vi "SMU_gate_2_sweep.vi"() -> ()   [LabVIEW 2022 SP3]
uses:
  Agilent U2722/Public/Configure/Configure Channel (Current).vi
  <vilib>/Analysis/1siggen.llb/Ramp Pattern by Delta.vi
  Agilent U2722/Public/Configure/Configure Channel (Voltage).vi
  Agilent U2722/Public/Data/Read Output (Single).vi
  <vilib>/Utility/file.llb/Write Delimited Spreadsheet (DBL).vi
  Agilent U2722/Agilent U2722.lvlib
  <vilib>/Analysis/NI_AALBase.lvlib
panel:
  in  "Tab Control":enum32{"Device Setup"}(tab)
  in  "OK Button":bool
  in  "Select Waveform":u16(ring) items=["Constant", "Sweep", "Pulse"]
  out "Vdd (V)":dbl
  in  "Voltage Range 2":u16(ring) items=["2 Volts", "20 Volts"]
  in  "Current Range 2":u16(ring)=4 items=["1 uA", "10 uA", "100 uA", "1 mA", "10 mA", "120 mA"]
  in  "Current Limit  2":dbl=0.005 format="%#_2p"
  in  "Voltage Range":u16(ring) items=["2 Volts", "20 Volts"]
  in  "Starting Voltage (V)":dbl
  in  "Stopping Voltage (V)":dbl=1.0
  in  "Voltage Interval  (DV)":dbl format="%#_2g"
  in  "Current Range":u16(ring)=4 items=["1 uA", "10 uA", "100 uA", "1 mA", "10 mA", "120 mA"]
  in  "VISA resource name SMU 1":refnum<visa-resource-name>
  in  "Gate 1 Channel Config":u16(ring)=1 items=["Channel 1"=1, "Channel 2"=2, "Channel 3"=3]
  in  "PLC":i32
  in  "Current Limit":dbl=0.005 format="%#_2p"
  in  "Interval Time (s)":dbl=1.0 caption="Delay Time (s)"
  in  "Vdd Channel Config":u16(ring)=2 items=["Channel 1"=1, "Channel 2"=2, "Channel 3"=3]
  in  "output file path":path
  out "XY Graph":cluster{"Y":dbl[], "Y":dbl[]}[](graph)
  in  "VISA resource name SMU 2":refnum<visa-resource-name>
  in  "Voltage Range 3":u16(ring) items=["2 Volts", "20 Volts"]
  in  "Current Range 3":u16(ring)=4 items=["1 uA", "10 uA", "100 uA", "1 mA", "10 mA", "120 mA"]
  in  "Gate 2 Channel Config":u16(ring)=1 items=["Channel 1"=1, "Channel 2"=2, "Channel 3"=3]
  in  "PLC 2":i32
  in  "Current Limit  3":dbl=0.005 format="%#_2p"
  in  "Output Measure Channel Config":u16(ring)=2 items=["Channel 1"=1, "Channel 2"=2, "Channel 3"=3]
  out "Idd (A)":dbl
  in  "Starting Voltage (V)":dbl
  in  "Stopping Voltage (V)":dbl=1.0
  in  "Voltage Interval  (DV)":dbl format="%#_2g"
  in  "Gate 2 Voltage (V)":dbl
  out "I_gate2 (A)":dbl
  out "V_gate2 (V)":dbl
  out "V_gate1 (A)":dbl
  out "I_gate1 (A)":dbl
  in  "Gate 1 Voltage (V)":dbl
  in  "Select Waveform":u16(ring) items=["Constant", "Sweep", "Pulse"]
  in  "Vdd (V) 2":dbl
  in  "Voltage Interval  (DV)":dbl format="%#_2g"
  in  "Stopping Voltage (V)":dbl=1.0
  in  "Starting Voltage (V)":dbl
  in  "Select Waveform":u16(ring) items=["Constant", "Sweep", "Pulse"]
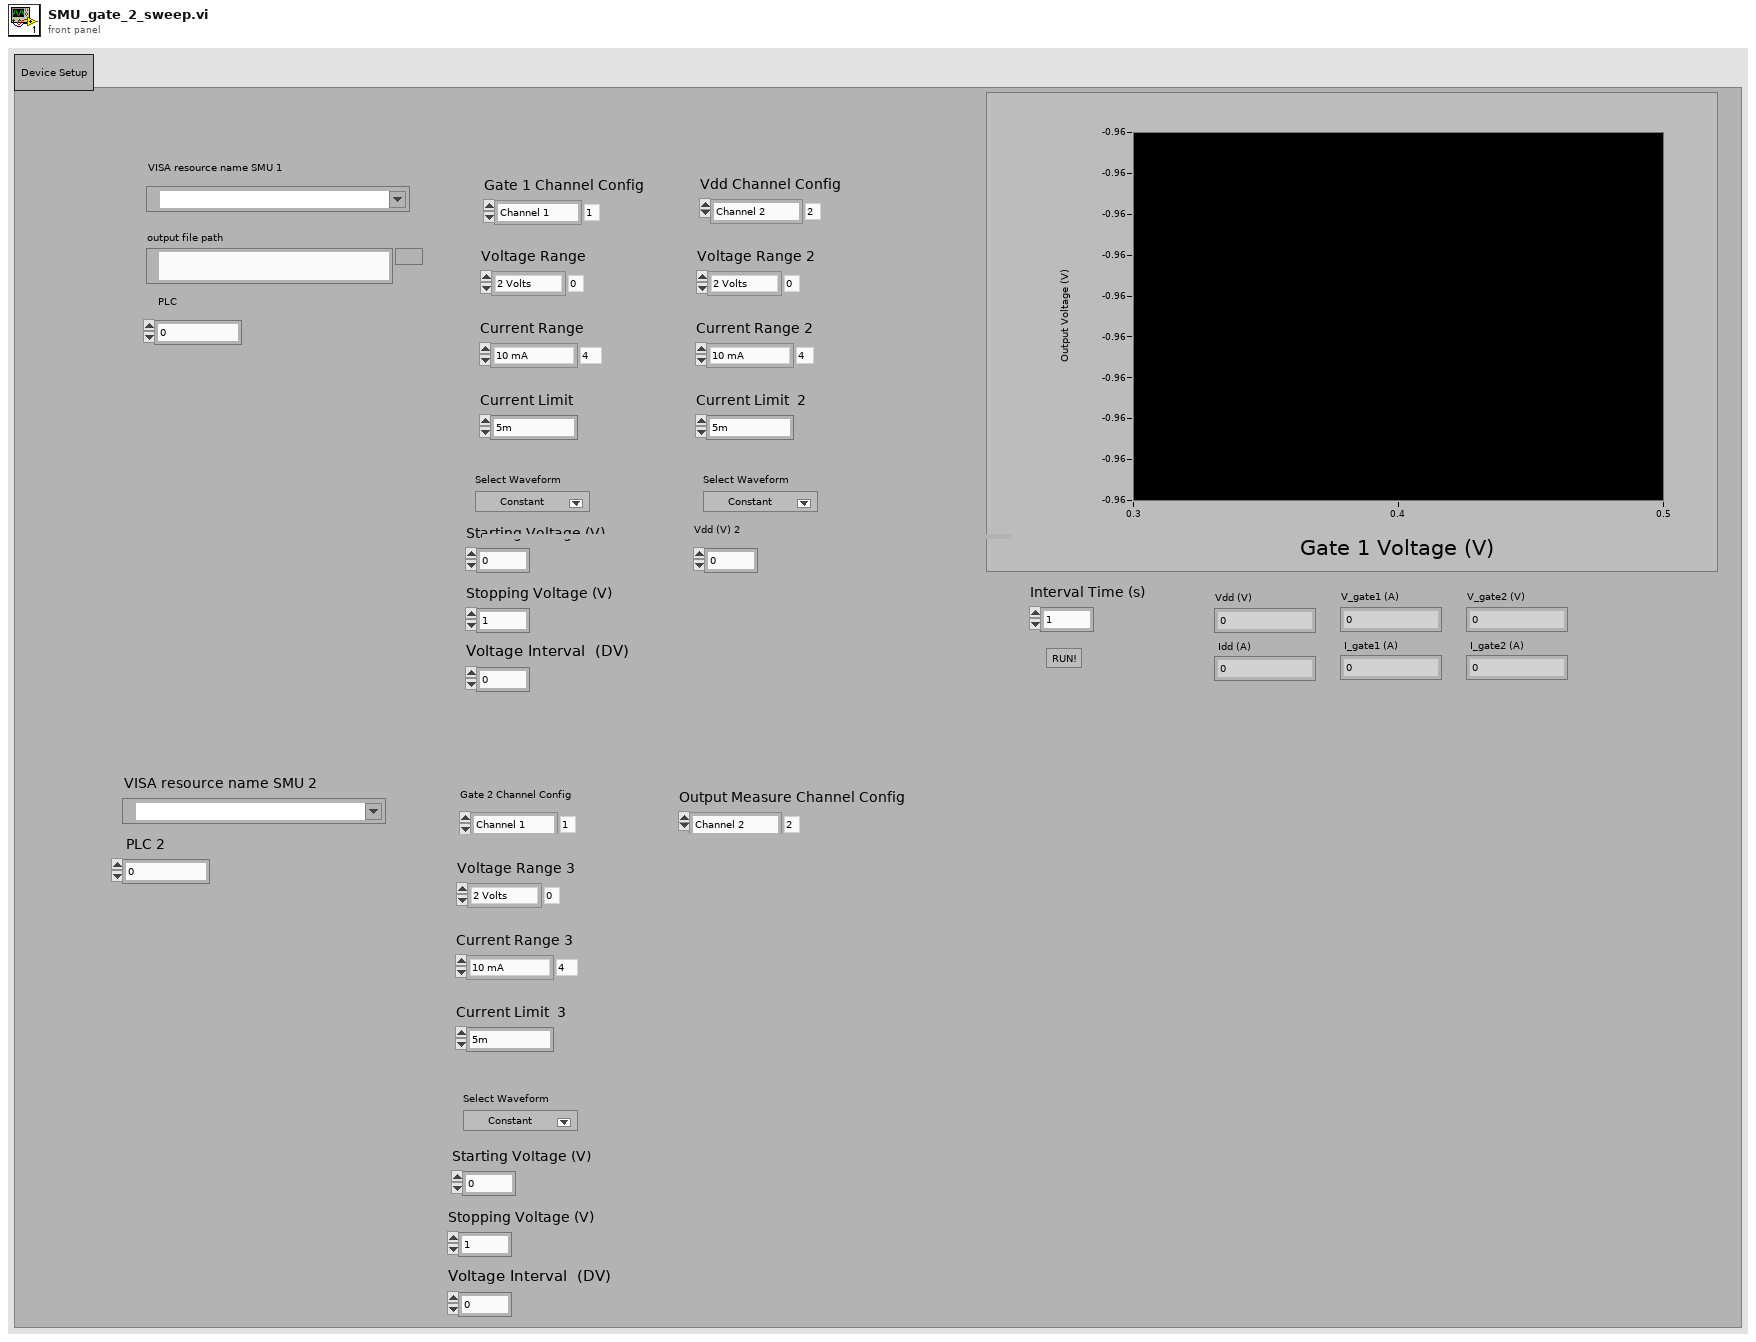
[diagram p1: front panel]
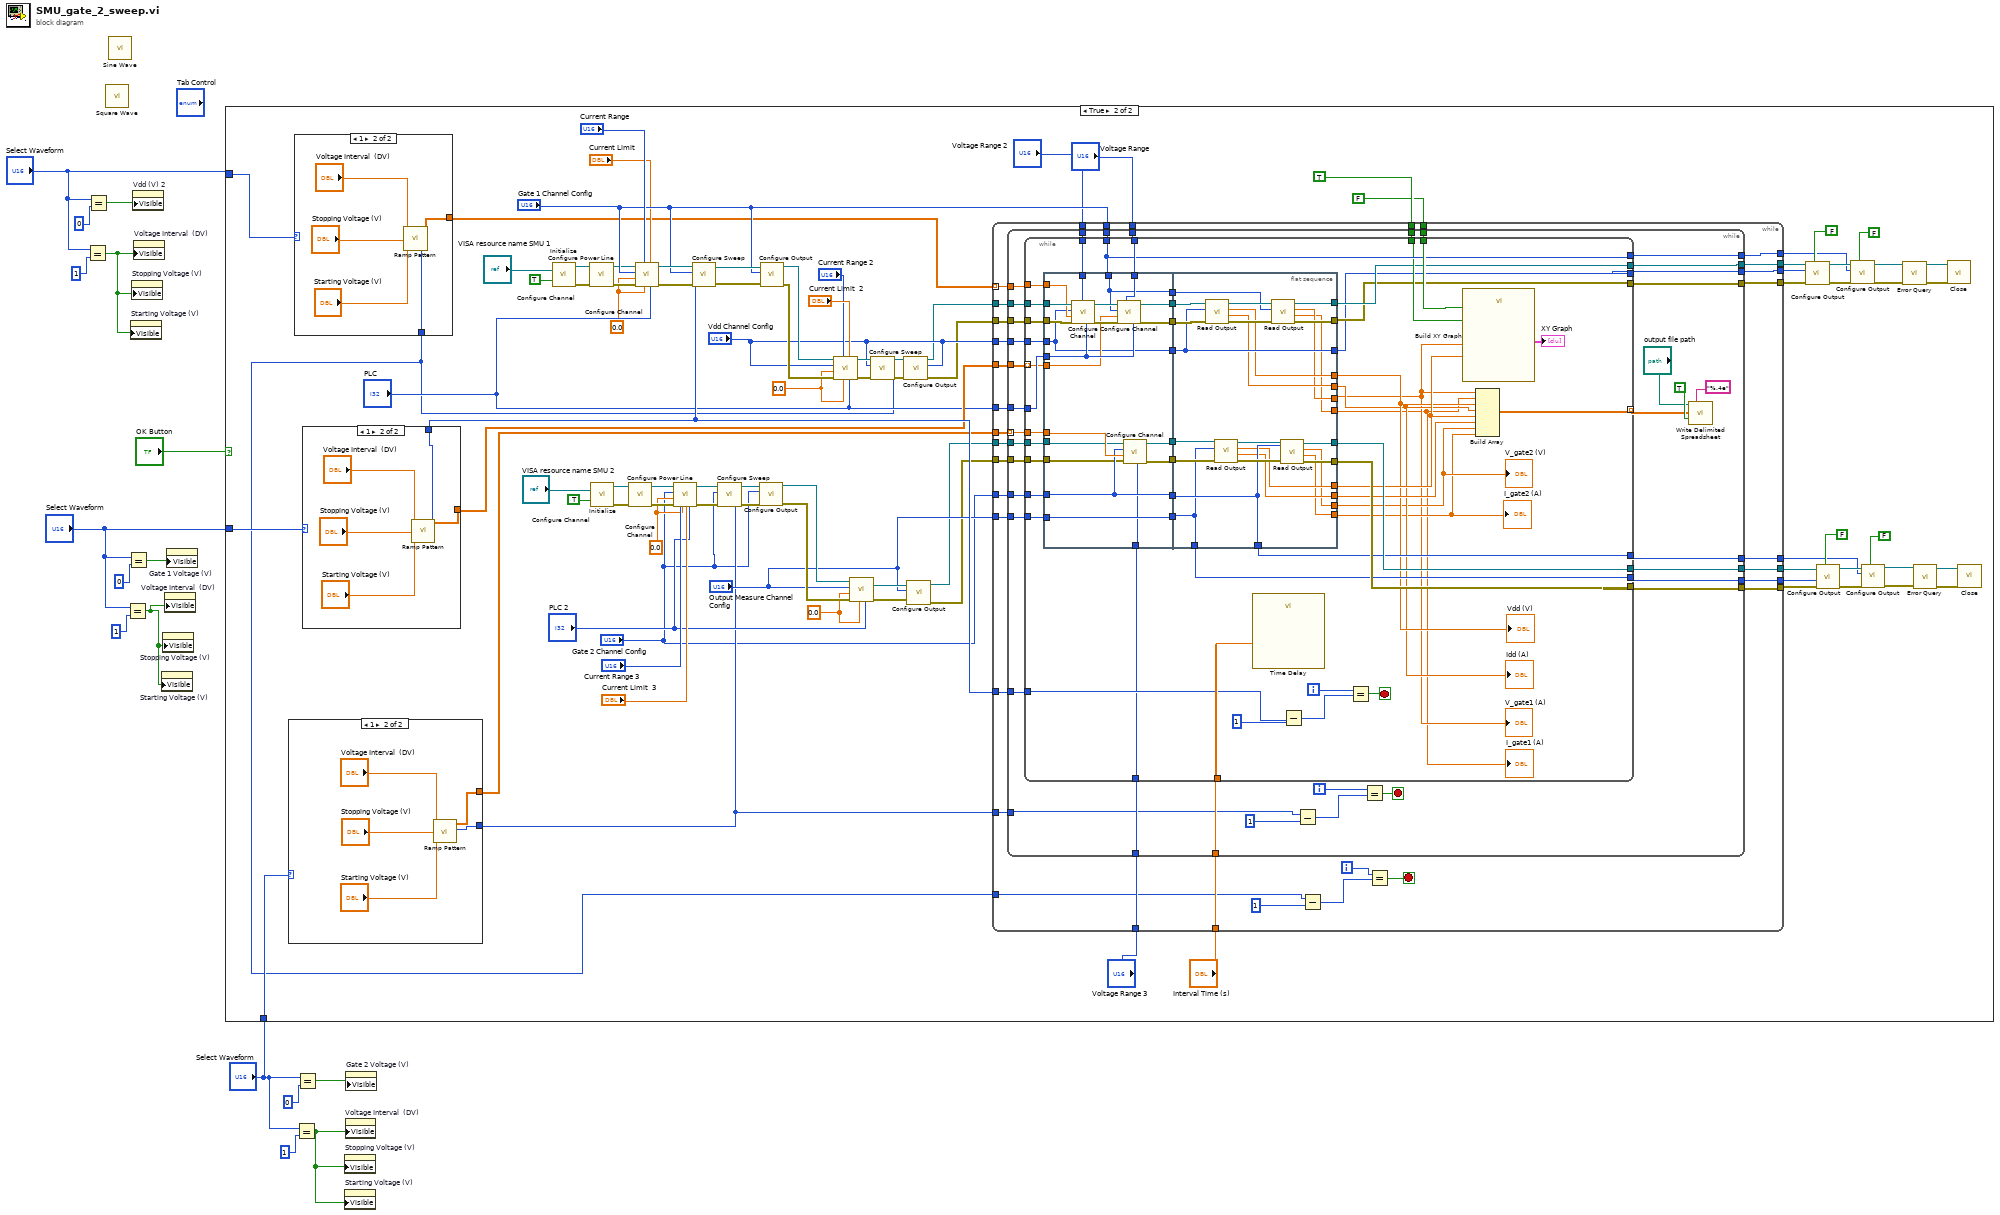
[diagram p0: block diagram]
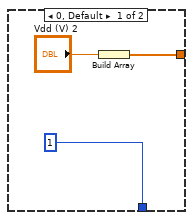
[diagram p3: hidden frame]
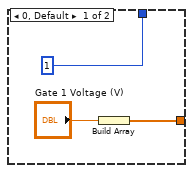
[diagram p4: hidden frame]
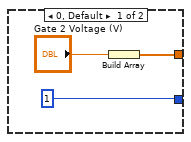
[diagram p5: hidden frame]
diagram:
  n1 = Equal?(x="Select Waveform", y=1) -> (x = y?=w3:bool)
  n2 = Equal?(x="Select Waveform", y=0) -> (x = y?=w2:bool)
  n3 = call <vilib>:"Square Wave.vi"() -> ()  [unwired: 6 in, 3 out]
  n4 = call <vilib>:"Sine Wave.vi"() -> ()  [unwired: 5 in, 3 out]
  n5 = Equal?(x="Select Waveform", y=1) -> (x = y?=w6:bool)
  n6 = Equal?(x="Select Waveform", y=0) -> (x = y?=w7:bool)
  n7 = property on="Starting Voltage (V)" class="DigNum (strict)"("Visible"=w3) -> ()  [unwired: 2 in, 2 out]
  n8 = property on="Stopping Voltage (V)" class="DigNum (strict)"("Visible"=w3) -> ()  [unwired: 2 in, 2 out]
  n9 = property on="Vdd (V) 2" class="DigNum (strict)"("Visible"=w2) -> ()  [unwired: 2 in, 2 out]
  n10 = property on="Voltage Interval  (DV)" class="DigNum (strict)"("Visible"=w3) -> ()  [unwired: 2 in, 2 out]
  n11 = property on="Starting Voltage (V)" class="DigNum (strict)"("Visible"=w6) -> ()  [unwired: 2 in, 2 out]
  n12 = property on="Stopping Voltage (V)" class="DigNum (strict)"("Visible"=w6) -> ()  [unwired: 2 in, 2 out]
  n13 = property on="Voltage Interval  (DV)" class="DigNum (strict)"("Visible"=w6) -> ()  [unwired: 2 in, 2 out]
  n14 = property on="Gate 1 Voltage (V)" class="DigNum (strict)"("Visible"=w7) -> ()  [unwired: 2 in, 2 out]
  n15 = case shown="True" "OK Button" {
    tunnel: "Select Waveform" -> [_ w38]
    tunnel: "Select Waveform" -> [_ w34]
    tunnel: "Select Waveform" -> [_ w33]
    frame False {
    }
    frame True {
      w58 = 0.0
      w57 = 0.0
      w71 = 0.0
      w70 = 0.0
      n16 = case shown="1" w38 {
        tunnel: [w285 w288] -> w37
        tunnel: [1 w287] -> w35
        frame 0, Default {
          n17 = Build Array("Gate 2 Voltage (V)") -> (w285:dbl[])
        }
        frame 1 {
          n18 = call-poly <vilib>:"Ramp Pattern.vi"("start"="Starting Voltage (V)", "end"="Stopping Voltage (V)", "delta"="Voltage Interval  (DV)") -> ("samples"=w287:i32, "Ramp Pattern"=w288:dbl[])  [unwired: 6 in, 1 out]
        }
      }
      n19 = case shown="1" w33 {
        tunnel: [1 w272] -> w26
        tunnel: [w268 w271] -> w28
        frame 0, Default {
          n20 = Build Array("Vdd (V) 2") -> (w268:dbl[])
        }
        frame 1 {
          n21 = call-poly <vilib>:"Ramp Pattern.vi"("start"="Starting Voltage (V)", "end"="Stopping Voltage (V)", "delta"="Voltage Interval  (DV)") -> ("samples"=w272:i32, "Ramp Pattern"=w271:dbl[])  [unwired: 6 in, 1 out]
        }
      }
      n22 = case shown="1" w34 {
        tunnel: [1 w280] -> w93
        tunnel: [w276 w279] -> w87
        frame 0, Default {
          n23 = Build Array("Gate 1 Voltage (V)") -> (w276:dbl[])
        }
        frame 1 {
          n24 = call-poly <vilib>:"Ramp Pattern.vi"("start"="Starting Voltage (V)", "end"="Stopping Voltage (V)", "delta"="Voltage Interval  (DV)") -> ("samples"=w280:i32, "Ramp Pattern"=w279:dbl[])  [unwired: 6 in, 1 out]
        }
      }
      n25 = call "Initialize.vi"("ID Query (True)"=TRUE, "VISA resource name"="VISA resource name SMU 1") -> ("error out"=w103:errorcluster, "VISA resource name out"=w102:refnum<visa-resource-name>)  [unwired: 8 in]
      n26 = call "Configure Power Line.vi"("error in (no error)"=w103, "VISA resource name"=w102) -> ("error out"=w89:errorcluster, "VISA resource name out"=w85:refnum<visa-resource-name>)  [unwired: 8 in]
      n27 = call "Initialize.vi"("ID Query (True)"=TRUE, "VISA resource name"="VISA resource name SMU 2") -> ("error out"=w66:errorcluster, "VISA resource name out"=w65:refnum<visa-resource-name>)  [unwired: 8 in]
      n28 = call "Configure Power Line.vi"("error in (no error)"=w66, "VISA resource name"=w65) -> ("error out"=w64:errorcluster, "VISA resource name out"=w62:refnum<visa-resource-name>)  [unwired: 8 in]
      n29 = call-poly "Configure Channel.vi"("Power Line Cycles (0)"="PLC", "Current Limit (1.0 uA)"="Current Limit", "Triggered Level (1.0 mA)"=w70, "Current Range (0: 1 uA)"="Current Range", "error in (no error)"=w89, "Output Level (1.0 mA)"=w70, "Channel (1: Channel 1)"="Gate 1 Channel Config", "VISA resource name"=w85) -> ("error out"=w90:errorcluster, "VISA resource name out"=w91:refnum<visa-resource-name>)  [unwired: 2 in]
      n30 = call-poly "Configure Channel.vi"("Power Line Cycles (0)"="PLC 2", "Current Limit (1.0 uA)"="Current Limit  3", "Triggered Level (1.0 mA)"=w57, "Current Range (0: 1 uA)"="Current Range 3", "error in (no error)"=w64, "Output Level (1.0 mA)"=w57, "Channel (1: Channel 1)"="Gate 2 Channel Config", "VISA resource name"=w62) -> ("error out"=w41:errorcluster, "VISA resource name out"=w42:refnum<visa-resource-name>)  [unwired: 2 in]
      n31 = call "Configure Sweep.vi"("error in (no error)"=w90, "Sweep Points (1)"=w93, "Channel (1: Channel 1)"="Gate 1 Channel Config", "VISA resource name"=w91) -> ("error out"=w94:errorcluster, "VISA resource name out"=w95:refnum<visa-resource-name>)  [unwired: 6 in]
      n32 = call "Configure Sweep.vi"("error in (no error)"=w41, "Sweep Points (1)"=w35, "Channel (1: Channel 1)"="Gate 2 Channel Config", "VISA resource name"=w42) -> ("error out"=w39:errorcluster, "VISA resource name out"=w40:refnum<visa-resource-name>)  [unwired: 6 in]
      n33 = call "Configure Output.vi"("error in (no error)"=w39, "Channel (1: Channel 1)"="Gate 2 Channel Config", "VISA resource name"=w40) -> ("error out"=w60:errorcluster, "VISA resource name out"=w61:refnum<visa-resource-name>)  [unwired: 7 in]
      n34 = call "Configure Output.vi"("error in (no error)"=w94, "Channel (1: Channel 1)"="Gate 1 Channel Config", "VISA resource name"=w95) -> ("error out"=w83:errorcluster, "VISA resource name out"=w84:refnum<visa-resource-name>)  [unwired: 7 in]
      n35 = call-poly "Configure Channel.vi"("Power Line Cycles (0)"="PLC", "Current Limit (1.0 uA)"="Current Limit  2", "Triggered Level (1.0 mA)"=w71, "Current Range (0: 1 uA)"="Current Range 2", "error in (no error)"=w83, "Output Level (1.0 mA)"=w71, "Channel (1: Channel 1)"="Vdd Channel Config", "VISA resource name"=w84) -> ("error out"=w29:errorcluster, "VISA resource name out"=w32:refnum<visa-resource-name>)  [unwired: 2 in]
      n36 = call-poly "Configure Channel.vi"("Power Line Cycles (0)"="PLC 2", "Triggered Level (1.0 mA)"=w58, "error in (no error)"=w60, "Output Level (1.0 mA)"=w58, "Channel (1: Channel 1)"="Output Measure Channel Config", "VISA resource name"=w61) -> ("error out"=w55:errorcluster, "VISA resource name out"=w56:refnum<visa-resource-name>)  [unwired: 4 in]
      n37 = call "Configure Sweep.vi"("error in (no error)"=w29, "Sweep Points (1)"=w26, "Channel (1: Channel 1)"="Vdd Channel Config", "VISA resource name"=w32) -> ("error out"=w30:errorcluster, "VISA resource name out"=w31:refnum<visa-resource-name>)  [unwired: 6 in]
      n38 = call "Configure Output.vi"("error in (no error)"=w30, "Channel (1: Channel 1)"="Vdd Channel Config", "VISA resource name"=w31) -> ("error out"=w25:errorcluster, "VISA resource name out"=w24:refnum<visa-resource-name>)  [unwired: 7 in]
      n39 = call "Configure Output.vi"("error in (no error)"=w55, "Channel (1: Channel 1)"="Output Measure Channel Config", "VISA resource name"=w56) -> ("error out"=w19:errorcluster, "VISA resource name out"=w20:refnum<visa-resource-name>)  [unwired: 7 in]
      n40 = while {
        tunnel: TRUE -> [w138]
        tunnel: FALSE -> [w137]
        tunnel: "Interval Time (s)" -> [w136]
        tunnel: w93 -> [w135]
        tunnel: "Voltage Range" -> [w134]
        tunnel: w87 -> [w133]
        tunnel: "Gate 1 Channel Config" -> [w132]
        tunnel: [w131] -> w77
        tunnel: [w130] -> w76
        tunnel: "PLC" -> [w129]
        tunnel: "Voltage Range 2" -> [w128]
        tunnel: "Output Measure Channel Config" -> [w127]
        tunnel: [w126] -> w45
        tunnel: [w125] -> w44
        tunnel: "Voltage Range 3" -> [w124]
        tunnel: w37 -> [w123]
        tunnel: w35 -> [w122]
        tunnel: "Gate 2 Channel Config" -> [w121]
        tunnel: w28 -> [w120] mode=indexing
        tunnel: "Vdd Channel Config" -> [w119]
        tunnel: w26 -> [w115]
        tunnel: w25 -> [w113]
        tunnel: w24 -> [w112]
        tunnel: [w111] -> w23
        tunnel: [w110] -> w22
        tunnel: w20 -> [w109]
        tunnel: w19 -> [w108]
        tunnel: [w107] -> w18
        tunnel: [w106] -> w17
        i -> [w116]
        stop <- w114 stop-if-true
        n41 = while {
          tunnel: w138 -> [w174]
          tunnel: w137 -> [w173]
          tunnel: w136 -> [w172]
          tunnel: w135 -> [w171]
          tunnel: w134 -> [w170]
          tunnel: w133 -> [w169]
          tunnel: w119 -> [w168]
          tunnel: w132 -> [w167]
          tunnel: [w166] -> w131
          tunnel: [w165] -> w130
          tunnel: w129 -> [w164]
          tunnel: w128 -> [w163]
          tunnel: w120 -> [w159]
          tunnel: w127 -> [w150]
          tunnel: [w158] -> w126
          tunnel: [w157] -> w125
          tunnel: w124 -> [w156]
          tunnel: w121 -> [w151]
          tunnel: w123 -> [w154] mode=indexing
          tunnel: w109 -> [w153]
          tunnel: w108 -> [w152]
          tunnel: w122 -> [w145]
          tunnel: [w144] -> w107
          tunnel: [w143] -> w106
          tunnel: w112 -> [w142]
          tunnel: w113 -> [w141]
          tunnel: [w140] -> w110
          tunnel: [w139] -> w111
          i -> [w147]
          stop <- w146 stop-if-true
          n42 = while {
            tunnel: w171 -> [w220]
            tunnel: w172 -> [w219]
            tunnel: w164 -> [w204]
            tunnel: w174 -> [w198]
            tunnel: w173 -> [w214]
            tunnel: [w197] -> w139
            tunnel: [w196] -> w140
            tunnel: w168 -> [w209]
            tunnel: w170 -> [w206]
            tunnel: w159 -> [w208]
            tunnel: [w215] -> w155 mode=indexing
            tunnel: w169 -> [w203] mode=indexing
            tunnel: w167 -> [w205]
            tunnel: w142 -> [w211]
            tunnel: [w195] -> w166
            tunnel: [w205] -> w165
            tunnel: w141 -> [w210]
            tunnel: w163 -> [w207]
            tunnel: [w194] -> w144
            tunnel: [w193] -> w143
            tunnel: w154 -> [w192]
            tunnel: [w189] -> w158
            tunnel: [w188] -> w157
            tunnel: w156 -> [w187]
            tunnel: w153 -> [w182]
            tunnel: w152 -> [w181]
            tunnel: w151 -> [w180]
            tunnel: w150 -> [w179]
            i -> [w217]
            stop <- w218 stop-if-true
            n43 = flat-sequence {
              tunnel: [w242] -> w213
              tunnel: [w240] -> w212
              tunnel: w211 -> [w239]
              tunnel: w210 -> [w238]
              tunnel: w209 -> [w232]
              tunnel: w208 -> [w237]
              tunnel: w207 -> [w236]
              tunnel: w206 -> [w235]
              tunnel: w205 -> [w231]
              tunnel: w204 -> [w234]
              tunnel: w203 -> [w233]
              tunnel: [w232] -> w202
              tunnel: [w231] -> w201
              tunnel: [w230] -> w200
              tunnel: [w229] -> w199
              tunnel: w182 -> [w224]
              tunnel: w181 -> [w223]
              tunnel: w179 -> [w227]
              tunnel: w192 -> [w228]
              tunnel: [w227] -> w191
              tunnel: w180 -> [w226]
              tunnel: [w226] -> w190
              tunnel: w187 -> [w225]
              tunnel: w213 -> [w267]
              tunnel: [w265] -> w197
              tunnel: w212 -> [w264]
              tunnel: [w262] -> w196
              tunnel: w202 -> [w254]
              tunnel: w201 -> [w261]
              tunnel: w200 -> [w260]
              tunnel: w199 -> [w258]
              tunnel: [w256] -> w194
              tunnel: [w255] -> w193
              tunnel: [w254] -> w195
              tunnel: w191 -> [w252]
              tunnel: w190 -> [w253]
              tunnel: [w253] -> w189
              tunnel: [w252] -> w188
              tunnel: [w251] -> w184
              tunnel: [w250] -> w183
              tunnel: [w249] -> w176
              tunnel: [w248] -> w175
              tunnel: [w247] -> w186
              tunnel: [w246] -> w185
              tunnel: [w245] -> w178
              tunnel: [w244] -> w177
              frame #0 {
                n44 = call-poly "Configure Channel.vi"("Power Line Cycles (0)"=w234, "Voltage Range (0: 2 Volts)"=w236, "error in (no error)"=w238, "Output Level (1.0 V)"=w237, "Channel (1: Channel 1)"=w232, "VISA resource name"=w239) -> ("error out"=w241:errorcluster, "VISA resource name out"=w243:refnum<visa-resource-name>)  [unwired: 4 in]
                n45 = call-poly "Configure Channel.vi"("Power Line Cycles (0)"=w234, "Voltage Range (0: 2 Volts)"=w235, "error in (no error)"=w241, "Output Level (1.0 V)"=w233, "Channel (1: Channel 1)"=w231, "VISA resource name"=w243) -> ("error out"=w240:errorcluster, "VISA resource name out"=w242:refnum<visa-resource-name>)  [unwired: 4 in]
                n46 = call-poly "Configure Channel.vi"("Voltage Range (0: 2 Volts)"=w225, "error in (no error)"=w223, "Output Level (1.0 V)"=w228, "Channel (1: Channel 1)"=w226, "VISA resource name"=w224) -> ("error out"=w229:errorcluster, "VISA resource name out"=w230:refnum<visa-resource-name>)  [unwired: 5 in]
              }
              frame #1 {
                n47 = call-poly "Read Output.vi"("error in (no error)"=w264, "Channel (1: Channel 1)"=w254, "VISA resource name"=w267) -> ("error out"=w263:errorcluster, "Actual Current Level (A)"=w250:dbl, "Actual Voltage Level (V)"=w251:dbl, "VISA resource name out"=w266:refnum<visa-resource-name>)  [unwired: 5 in]
                n48 = call-poly "Read Output.vi"("error in (no error)"=w258, "Channel (1: Channel 1)"=w252, "VISA resource name"=w260) -> ("error out"=w257:errorcluster, "Actual Current Level (A)"=w246:dbl, "Actual Voltage Level (V)"=w247:dbl, "VISA resource name out"=w259:refnum<visa-resource-name>)  [unwired: 5 in]
                n49 = call-poly "Read Output.vi"("error in (no error)"=w263, "Channel (1: Channel 1)"=w261, "VISA resource name"=w266) -> ("error out"=w262:errorcluster, "Actual Current Level (A)"=w248:dbl, "Actual Voltage Level (V)"=w249:dbl, "VISA resource name out"=w265:refnum<visa-resource-name>)  [unwired: 5 in]
                n50 = call-poly "Read Output.vi"("error in (no error)"=w257, "Channel (1: Channel 1)"=w253, "VISA resource name"=w259) -> ("error out"=w255:errorcluster, "Actual Current Level (A)"=w244:dbl, "Actual Voltage Level (V)"=w245:dbl, "VISA resource name out"=w256:refnum<visa-resource-name>)  [unwired: 5 in]
              }
            }
            n51 = call "Time Delay"("Delay Time (s)"=w219) -> ()  [unwired: 10 in, 1 out]
            n52 = Subtract(x=w220, y=1 ("x")) -> (x-y=w221:i32)
            n53 = Equal?(x=w217, y=w221) -> (x = y?=w218:bool)
            n54 = call "Build XY Graph"("Enable"=w198, "Reset"=w214, "Y Input"=w186, "X Input"=w176) -> ("XY Graph"=→"XY Graph":cluster{"X":dbl[], "Y":dbl[]}[])  [unwired: 6 in, 1 out]
            n55 = Build Array(w176, w175, w184, w183, w186, w185, w178, w177) -> (w215:dbl[])
            "Vdd (V)" <- w184
            "Idd (A)" <- w183
            "V_gate2 (V)" <- w178
            "I_gate2 (A)" <- w177
            "V_gate1 (A)" <- w176
            "I_gate1 (A)" <- w175
          }
          n56 = Subtract(x=w145, y=1 ("x")) -> (x-y=w148:i32)
          n57 = Equal?(x=w147, y=w148) -> (x = y?=w146:bool)
          n58 = call-poly <vilib>:"Write Delimited Spreadsheet.vi"("file path (dialog if empty)"="output file path", "format (%.3f)"="%.4e", "2D data"=w155, "append to file? (new file:F)"=TRUE) -> ()  [unwired: 10 in, 2 out]
        }
        n59 = Subtract(x=w115, y=1 ("x")) -> (x-y=w117:i32)
        n60 = Equal?(x=w116, y=w117) -> (x = y?=w114:bool)
      }
      n61 = call "Configure Output.vi"("Enable Output (T: Enable)"=FALSE, "error in (no error)"=w22, "Channel (1: Channel 1)"=w77, "VISA resource name"=w23) -> ("error out"=w80:errorcluster, "VISA resource name out"=w82:refnum<visa-resource-name>)  [unwired: 6 in]
      n62 = call "Configure Output.vi"("Enable Output (T: Enable)"=FALSE, "error in (no error)"=w17, "Channel (1: Channel 1)"=w44, "VISA resource name"=w18) -> ("error out"=w49:errorcluster, "VISA resource name out"=w51:refnum<visa-resource-name>)  [unwired: 6 in]
      n63 = call "Configure Output.vi"("Enable Output (T: Enable)"=FALSE, "error in (no error)"=w80, "Channel (1: Channel 1)"=w76, "VISA resource name"=w82) -> ("error out"=w79:errorcluster, "VISA resource name out"=w81:refnum<visa-resource-name>)  [unwired: 6 in]
      n64 = call "Configure Output.vi"("Enable Output (T: Enable)"=FALSE, "error in (no error)"=w49, "Channel (1: Channel 1)"=w45, "VISA resource name"=w51) -> ("error out"=w48:errorcluster, "VISA resource name out"=w50:refnum<visa-resource-name>)  [unwired: 6 in]
      n65 = call "Error Query.vi"("error in (no error)"=w79, "VISA resource name"=w81) -> ("error out"=w97:errorcluster, "VISA resource name out"=w96:refnum<visa-resource-name>)  [unwired: 6 in, 2 out]
      n66 = call "Error Query.vi"("error in (no error)"=w48, "VISA resource name"=w50) -> ("error out"=w53:errorcluster, "VISA resource name out"=w52:refnum<visa-resource-name>)  [unwired: 6 in, 2 out]
      n67 = call "Close.vi"("error in (no error)"=w97, "VISA resource name"=w96) -> ()  [unwired: 9 in, 1 out]
      n68 = call "Close.vi"("error in (no error)"=w53, "VISA resource name"=w52) -> ()  [unwired: 9 in, 1 out]
    }
  }
  n69 = Equal?(x="Select Waveform", y=1) -> (x = y?=w11:bool)
  n70 = Equal?(x="Select Waveform", y=0) -> (x = y?=w14:bool)
  n71 = property on="Stopping Voltage (V)" class="DigNum (strict)"("Visible"=w11) -> ()  [unwired: 2 in, 2 out]
  n72 = property on="Starting Voltage (V)" class="DigNum (strict)"("Visible"=w11) -> ()  [unwired: 2 in, 2 out]
  n73 = property on="Voltage Interval  (DV)" class="DigNum (strict)"("Visible"=w11) -> ()  [unwired: 2 in, 2 out]
  n74 = property on="Gate 2 Voltage (V)" class="DigNum (strict)"("Visible"=w14) -> ()  [unwired: 2 in, 2 out]
